vi "1B_AppendArray.vi"(2 "append":dbl, 3 "Array":dbl[](array[numeric])) -> (1 "Array out":dbl[](array[numeric]))   [LabVIEW 2010]
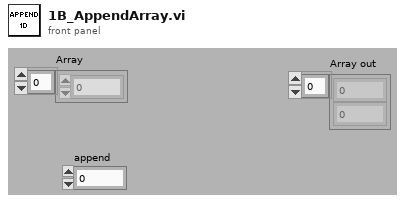
[diagram p1: front panel]
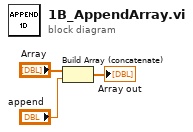
[diagram p0: block diagram]
diagram:
  n1 = Build Array (concatenate)("Array", "append") -> (→"Array out":dbl[])
